vi "XML Cluster.vi"() -> ()   [LabVIEW 2016]
panel:
  out "Configuration Properties 2":T1
  in  "Configuration Properties":T2
  out "xml string":string
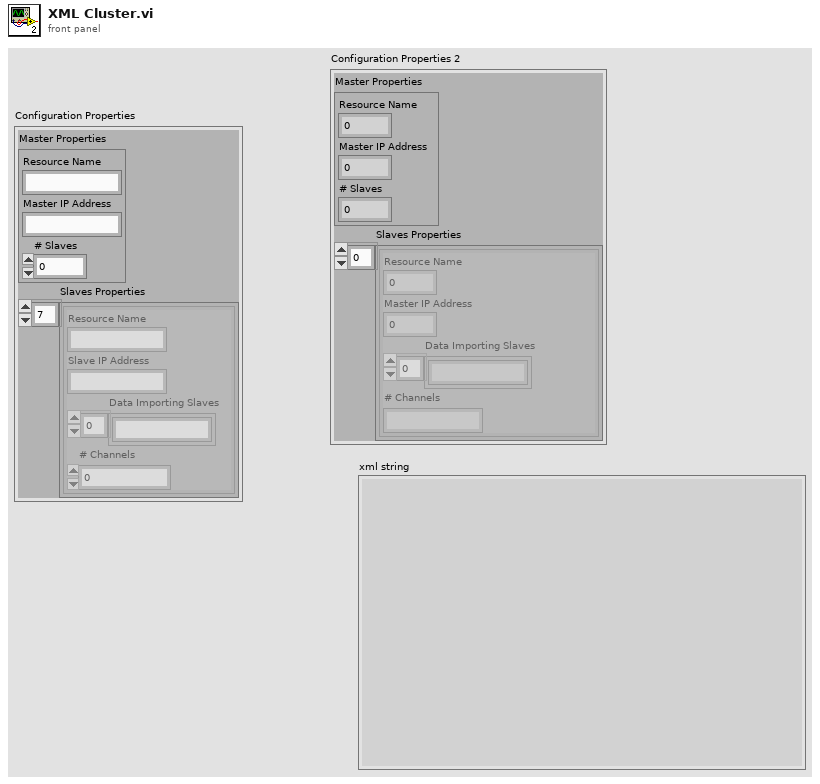
[diagram p1: front panel]
types:
  T1 = cluster{"Master Properties":cluster{"Resource Name":dbl, "Master IP Address":dbl, "# Slaves":dbl}, "Slaves Properties":cluster{"Resource Name":dbl, "Master IP Address":dbl, "Data Importing Slaves":string[], "# Channels":string}[]}
  T2 = cluster{"Master Properties":cluster{"Resource Name":string, "Master IP Address":string, "# Slaves":dbl}, "Slaves Properties":cluster{"Resource Name":string, "Slave IP Address":string, "Data Importing Slaves":string[], "# Channels":dbl}[]}
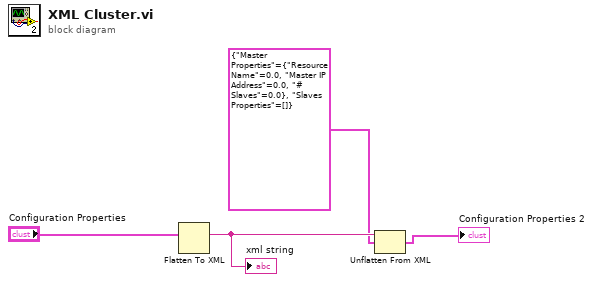
[diagram p0: block diagram]
diagram:
  n1 = Flatten To XML(anything="Configuration Properties") -> (xml string=w4:string)
  "xml string" <- w4
  n2 = Unflatten From XML(xml string=w4, type=T1 {"Master Properties"={"Resource Name"=0.0, "Master IP Address"=0.0, "# Slaves"=0.0}, "Slaves Properties"=[]} ("Configuration Properties")) -> (value=→"Configuration Properties 2":T1)  [unwired: 1 in, 1 out]
